vi "Profile B Generation v1.vi"() -> ()   [LabVIEW 2018]
uses:
  <vilib>/Utility/file.llb/Write Delimited Spreadsheet (DBL).vi
  <vilib>/addons/Time Series Analysis/Statistical Analysis.llb/TSA Normal Distribution Test (Array).vi
  <vilib>/express/express analysis/Spectral/Block/exnSpectralBlock spectral measurements power poly.vi
  <vilib>/express/express analysis/Spectral/Block/exnSpectralBlock spectral measurements power WFM.vi
  <vilib>/express/express analysis/Spectral/XNode/ExpressSpectralMeasurementsBlockNode.xnode
  <vilib>/addons/_Advanced Signal Processing/NI_AdvSigProcTSA.lvlib
  <vilib>/measure/NI_MABase.lvlib
panel:
  in  "filter specifications":T1={"lower cutoff freq"=0.1, "higher cutoff freq"=2.0, "order"=5}
  in  "Standard Deviation":dbl=0.0009148153893115104
  in  "exponent 2":dbl=0.8 format="%.2p"
  in  "noise density":dbl=0.47 format="%.2p"
  out "Power Spectrum (Hanning window)":cluster{"f0":dbl, "df":dbl, "magnitude":dbl[]}(graph)
  out "Histogram":cluster{"Axis":dbl[], dbl[]}[](graph)
  out "Data":dbl[][](graph)
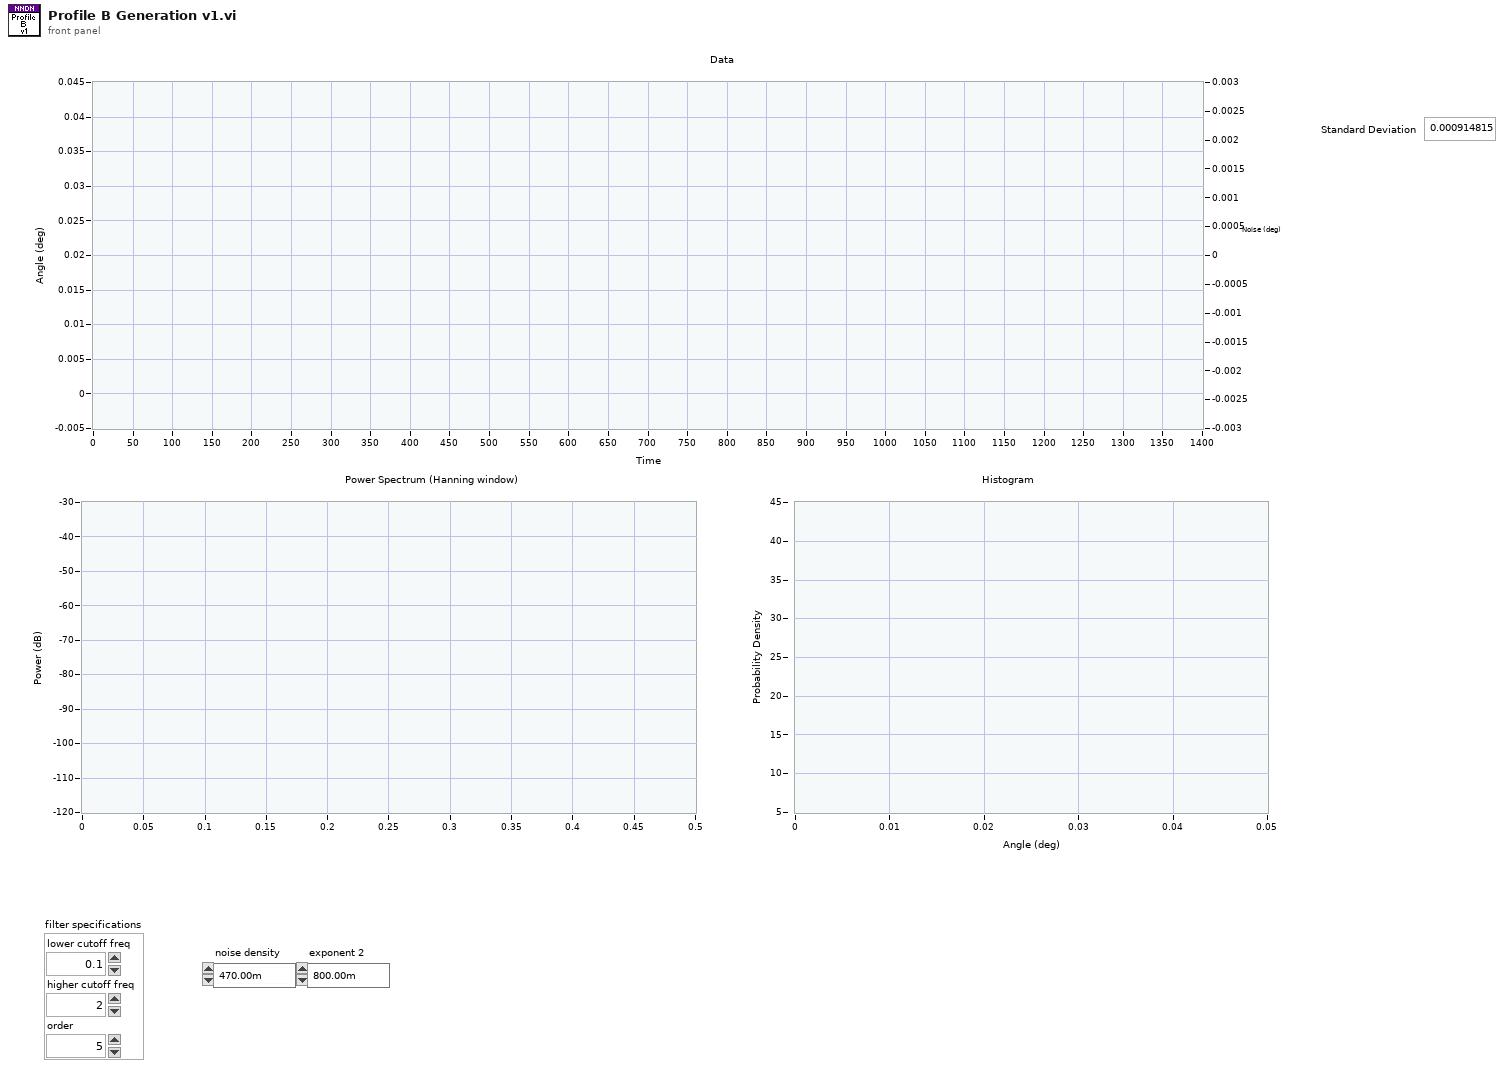
[diagram p1: front panel]
types:
  T1 = cluster{"lower cutoff freq":dbl, "higher cutoff freq":dbl, "order":i32}
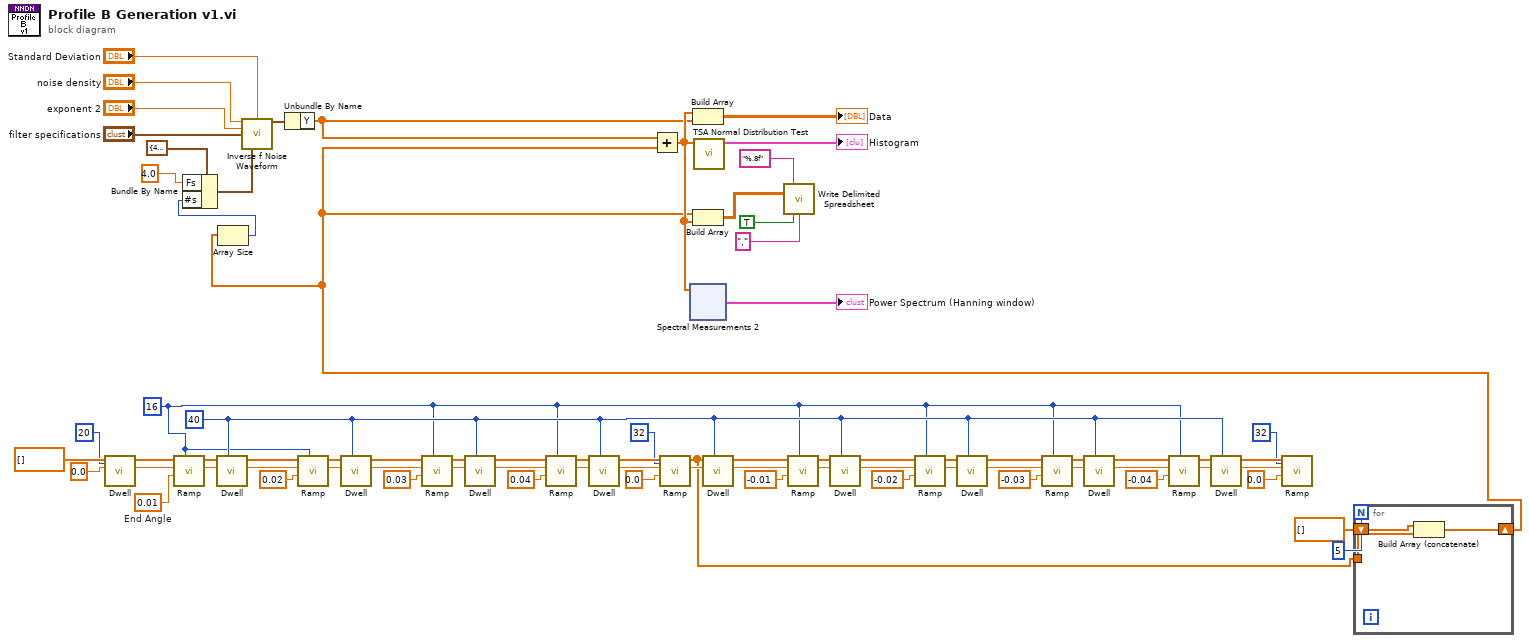
[diagram p0: block diagram]
diagram:
  w7 = 40 ("Points")
  w59 = 0.01  # End Angle
  w6 = 16
  n1 = call "Dwell.vi"("Points"=20, "Angle"=0.0, "Array In"=dbl[] [] ("Array Out")) -> ("Last Point"=w49:dbl, "Array Out"=w50:dbl[])  [unwired: 7 in]
  n2 = call "Ramp.vi"("Points"=w6, "End Angle"=w59, "Start Angle"=w49, "Array In"=w50) -> ("Last Value"=w57:dbl, "Array Out"=w58:dbl[])  [unwired: 6 in]
  n3 = call "Dwell.vi"("Points"=w7, "Angle"=w57, "Array In"=w58) -> ("Last Point"=w55:dbl, "Array Out"=w56:dbl[])  [unwired: 7 in]
  n4 = call "Ramp.vi"("Points"=w6, "End Angle"=0.02, "Start Angle"=w55, "Array In"=w56) -> ("Last Value"=w44:dbl, "Array Out"=w45:dbl[])  [unwired: 6 in]
  n5 = call "Dwell.vi"("Points"=w7, "Angle"=w44, "Array In"=w45) -> ("Last Point"=w47:dbl, "Array Out"=w46:dbl[])  [unwired: 7 in]
  n6 = call "Ramp.vi"("Points"=w6, "End Angle"=0.03, "Start Angle"=w47, "Array In"=w46) -> ("Last Value"=w42:dbl, "Array Out"=w43:dbl[])  [unwired: 6 in]
  n7 = call "Dwell.vi"("Points"=w7, "Angle"=w42, "Array In"=w43) -> ("Last Point"=w37:dbl, "Array Out"=w38:dbl[])  [unwired: 7 in]
  n8 = call "Ramp.vi"("Points"=w6, "End Angle"=0.04, "Start Angle"=w37, "Array In"=w38) -> ("Last Value"=w41:dbl, "Array Out"=w40:dbl[])  [unwired: 6 in]
  n9 = call "Dwell.vi"("Points"=w7, "Angle"=w41, "Array In"=w40) -> ("Last Point"=w35:dbl, "Array Out"=w36:dbl[])  [unwired: 7 in]
  n10 = call "Ramp.vi"("Points"=32, "End Angle"=0.0, "Start Angle"=w35, "Array In"=w36) -> ("Last Value"=w32:dbl, "Array Out"=w3:dbl[])  [unwired: 6 in]
  n11 = call "Dwell.vi"("Points"=w7, "Angle"=w32, "Array In"=w3) -> ("Last Point"=w31:dbl, "Array Out"=w30:dbl[])  [unwired: 7 in]
  n12 = call "Ramp.vi"("Points"=w6, "End Angle"=-0.01, "Start Angle"=w31, "Array In"=w30) -> ("Last Value"=w27:dbl, "Array Out"=w28:dbl[])  [unwired: 6 in]
  n13 = call "Dwell.vi"("Points"=w7, "Angle"=w27, "Array In"=w28) -> ("Last Point"=w16:dbl, "Array Out"=w17:dbl[])  [unwired: 7 in]
  n14 = call "Ramp.vi"("Points"=w6, "End Angle"=-0.02, "Start Angle"=w16, "Array In"=w17) -> ("Last Value"=w26:dbl, "Array Out"=w25:dbl[])  [unwired: 6 in]
  n15 = call "Dwell.vi"("Points"=w7, "Angle"=w26, "Array In"=w25) -> ("Last Point"=w14:dbl, "Array Out"=w15:dbl[])  [unwired: 7 in]
  n16 = call "Ramp.vi"("Points"=w6, "End Angle"=-0.03, "Start Angle"=w14, "Array In"=w15) -> ("Last Value"=w21:dbl, "Array Out"=w22:dbl[])  [unwired: 6 in]
  n17 = call "Dwell.vi"("Points"=w7, "Angle"=w21, "Array In"=w22) -> ("Last Point"=w12:dbl, "Array Out"=w13:dbl[])  [unwired: 7 in]
  n18 = call "Ramp.vi"("Points"=w6, "End Angle"=-0.04, "Start Angle"=w12, "Array In"=w13) -> ("Last Value"=w20:dbl, "Array Out"=w19:dbl[])  [unwired: 6 in]
  n19 = call "Dwell.vi"("Points"=w7, "Angle"=w20, "Array In"=w19) -> ("Last Point"=w10:dbl, "Array Out"=w11:dbl[])  [unwired: 7 in]
  n20 = call "Ramp.vi"("Points"=32, "End Angle"=0.0, "Start Angle"=w10, "Array In"=w11) -> ()  [unwired: 6 in, 2 out]
  n21 = for {
    N: 5 -> [_]
    tunnel: w3 -> [w79]
    shift-right: [w78] -> w2
    shift-left: dbl[] [] -> [w77]
    n22 = Build Array (concatenate)(w77, w79) -> (w78:dbl[])
  }
  n23 = Array Size(array=w2) -> (size(s)=w1:i32)
  n24 = Bundle By Name(cluster=cluster{"Fs":dbl, "#s":dbl} {"Fs"=4.0, "#s"=1000.0} ("sampling info"), "Fs"=4.0, "#s"=w1) -> (w65:cluster{"Fs":dbl, "#s":dbl})
  n25 = call <vilib>:"Inverse f Noise Waveform.vi"("noise density"="noise density", "standard deviation"="Standard Deviation", "exponent"="exponent 2", "filter specifications"="filter specifications", "sampling info"=w65) -> ("signal out"=w67:waveform(dbl))  [unwired: 6 in, 4 out]
  n26 = Unbundle By Name(w67) -> ("Y"=w60:dbl[])
  n27 = Add(x=w60, y=w2) -> (x+y=w62:dbl[])
  n28 = xnode "Spectral Measurements 2"("Signals"=w62) -> ("Power Spectrum"=→"Power Spectrum (Hanning window)":cluster{"f0":dbl, "df":dbl, "magnitude":dbl[]})  [unwired: 1 in, 1 out]
  n29 = Build Array(w62, w60) -> (→"Data":dbl[][])
  n30 = Build Array(w2, w62) -> (w61:dbl[][])
  n31 = call-poly <vilib>:"TSA Normal Distribution Test.vi"("Xt"=w62) -> ("histogram"=→"Histogram":cluster{"Axis":dbl[], dbl[]}[])  [unwired: 9 in, 1 out]
  n32 = call-poly <vilib>:"Write Delimited Spreadsheet.vi"("format (%.3f)"="%.8f", "2D data"=w61, "transpose? (no:F)"=TRUE, "delimiter (\\t)"="," ("delimiter (\\t)")) -> ()  [unwired: 10 in, 2 out]
